vi "End Preview.vi"(8 "error in (no error)":errorcluster, 10 "Preview":bool, 11 "GUI Interface in":refnum<class "GUI Interface.lvclass">) -> (0 "error out":errorcluster, 3 "GUI Interface out":refnum<class "GUI Interface.lvclass">)   [LabVIEW 2020, in "GUI.lvlib" / "GUI Interface.lvclass"]
uses:
  GUI Interface.lvclass
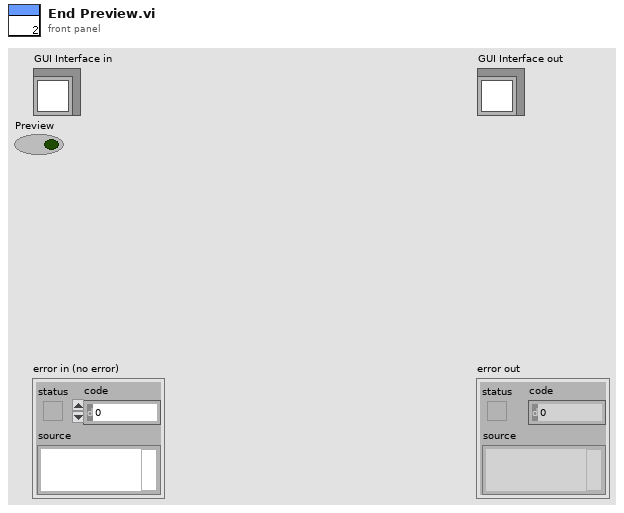
[diagram p1: front panel]
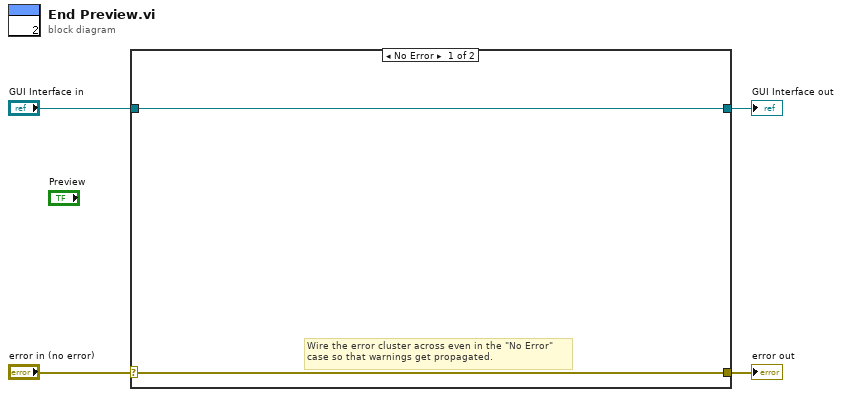
[diagram p0: block diagram]
diagram:
  n1 = case shown="No Error" "error in (no error)" {
    selector: "error in (no error)" -> [w5 w8]
    tunnel: [w5 w8] -> w3
    tunnel: [w6 w7] -> w1
    tunnel: "GUI Interface in" -> [w6 w7]
    frame No Error {
      # "Wire the error cluster across even in the \"No Error\"\ncase so that warnings get propagated."
    }
    frame Error {
    }
  }
  "error out" <- w3
  "GUI Interface out" <- w1
